vi "detectAllVarables.vi"(3 "error in (no error)":errorcluster, 5 "VISA resource name":refnum<visa-resource-name>="COM1" caption="端口号") -> (0 "error out":errorcluster, 1 "Data":T1[](array[typedef]), 2 "VISA resource name 2":refnum<visa-resource-name>="COM1" caption="端口号")   [LabVIEW 2010]
uses:
  OutputDataFormat.ctl
  VarableID.ctl
  AmmeterGlobalCostants.vi
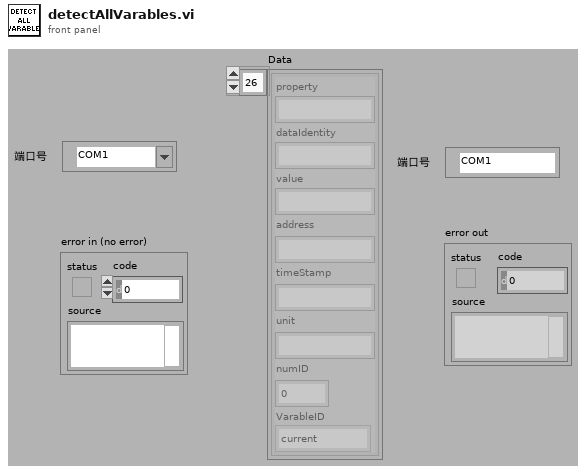
[diagram p1: front panel]
types:
  T1 = typedef "OutputDataFormat.ctl" = cluster{"property":string, "dataIdentity":string, "value":string, "address":string, "timeStamp":string, "unit":string, "numID":i32, "VarableID":T2}
  T2 = typedef "VarableID.ctl" = enum16{"current", "power", "PF", "voltage"}
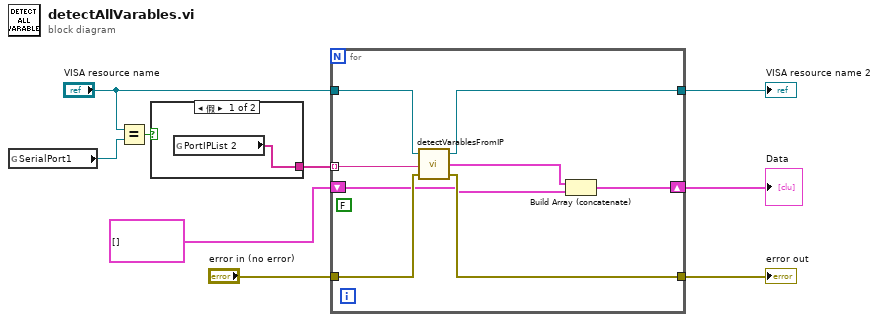
[diagram p0: block diagram]
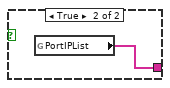
[diagram p2: hidden frame]
diagram:
  n1 = global read "AmmeterGlobalCostants.vi" "SerialPort1"() -> (w3:refnum<visa-resource-name>)
  n2 = Equal?(x="VISA resource name", y=w3) -> (x = y?=w1:bool)
  n3 = case shown="假" w1 {
    tunnel: [w10 w11] -> w6
    frame False {
      n4 = global read "AmmeterGlobalCostants.vi" "PortIPList 2"() -> (w10:string[])
    }
    frame True {
      n5 = global read "AmmeterGlobalCostants.vi" "PortIPList"() -> (w11:string[])
    }
  }
  n6 = for {
    tunnel: [w19] -> w9
    tunnel: [w18] -> w8
    tunnel: "error in (no error)" -> [w17]
    tunnel: "VISA resource name" -> [w16]
    tunnel: w6 -> [w15] mode=indexing
    shift-right: [w13] -> w5
    shift-left: T1[] [] -> [w12]
    (unwired) FALSE
    n7 = call "detectVarablesFromIP.vi"("error in (no error)"=w17, "PortIP"=w15, "VISA resource name"=w16) -> ("error out"=w18:errorcluster, "Data"=w14:T1[], "VISA resource name 2"=w19:refnum<visa-resource-name>)
    n8 = Build Array (concatenate)(w14, w12) -> (w13:T1[])
  }
  "VISA resource name 2" <- w9
  "error out" <- w8
  "Data" <- w5
